vi "Init.vi"(8 "error in (no error)":errorcluster, 11 "Bicycle in":refnum<class "Bicycle.lvclass">) -> (0 "error out":errorcluster, 3 "Bicycle out":refnum<class "Bicycle.lvclass">)   [LabVIEW 2019, in "Bicycle.lvclass"]
uses:
  Bicycle.lvclass
  Vehicle/Vehicle.lvclass/Vehicle.ctl
  Vehicle/Vehicle.lvclass
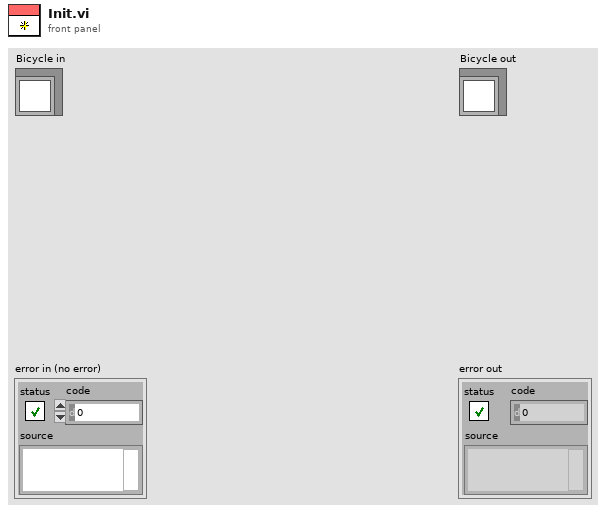
[diagram p1: front panel]
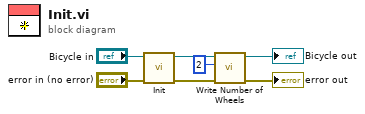
[diagram p0: block diagram]
diagram:
  n1 = call-parent "Init.vi"("error in (no error)"="error in (no error)", "Vehicle in"="Bicycle in") -> ("error out"=w5:errorcluster, "Vehicle out"=w4:refnum<class "Bicycle.lvclass">)  [unwired: 8 in]
  n2 = call "Write Number of Wheels .vi"("error in (no error)"=w5, "Number of Wheels"=2, "Vehicle in"=w4) -> ("error out"=→"error out":errorcluster, "Vehicle out"=→"Bicycle out":refnum<class "Bicycle.lvclass">)  [unwired: 7 in]
